vi "Utility Error Query.vi"(5 "Retry Attempts (0)":i32 min=0, 8 "error in (no error)":errorcluster, 11 "VISA resource name":refnum<visa-resource-name>) -> (0 "error out":errorcluster, 1 "Error Message":string, 2 "Error Code":i32[](array[numeric]), 3 "VISA resource name out":refnum<visa-resource-name>)   [LabVIEW 2020, in "ChromTech Series I Drivers.lvlib"]
doc: "Queries the instrument for any errors in the instrument's error queue. It will continue to read errors until all errors have been read from the instrument. Any errors will be returned in the <B>error out</B> control.\n\n<B>Note:</B>\nThis VI is called automatically by most driver VIs so it is not usually necessary to call this in an application."
uses:
  <instrlib>/RxnRover/ChromtechSeriesIDriver/ChromTech Series I Drivers.lvlib
panel:
  # "THIS IS NOT COMPLETE"
  # "EDIT: Note: The Error Query VI is included as a subVI in all driver VIs except low-level API VIs. If the instrument does not support error query, then remove the VI and remove subVI calls in each instrument driver VI that calls it."
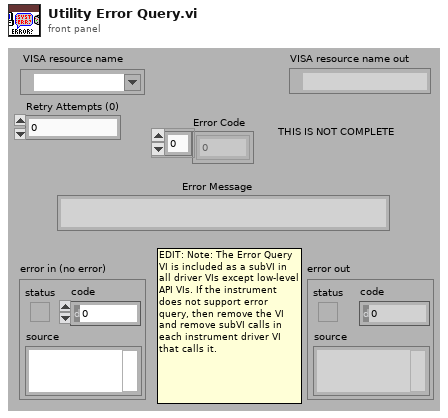
[diagram p1: front panel]
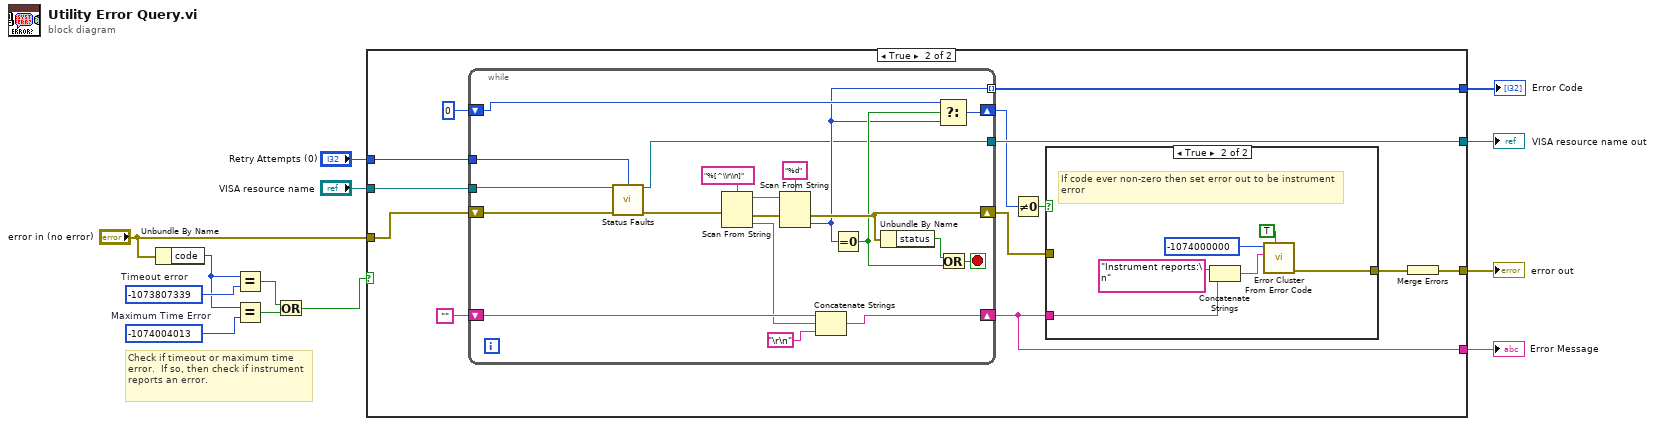
[diagram p0: block diagram]
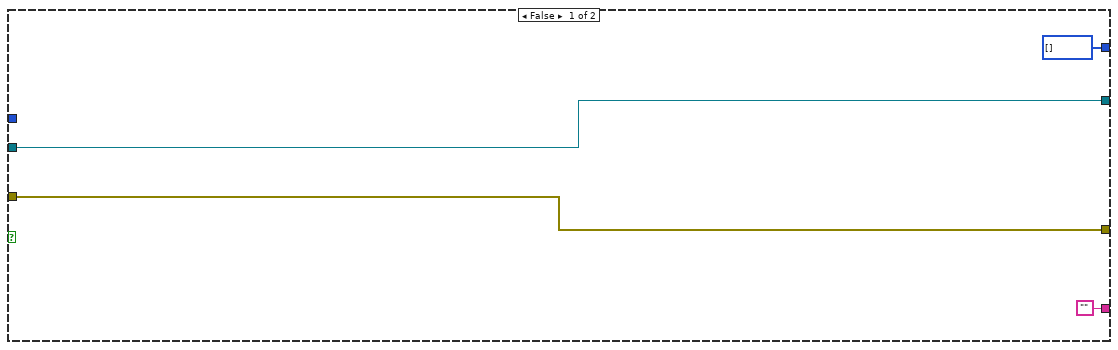
[diagram p2: hidden frame]
diagram:
  w6 = -1074004013  # Maximum Time Error
  w8 = -1073807339  # Timeout error
  # "Check if timeout or maximum time error.  If so, then check if instrument reports an error."
  n1 = Unbundle By Name("error in (no error)") -> ("code"=w7:i32)
  n2 = Equal?(x=w7, y=w8) -> (x = y?=w4:bool)
  n3 = Equal?(x=w7, y=w6) -> (x = y?=w5:bool)
  n4 = Or(x=w4, y=w5) -> (x .or. y?=w2:bool)
  n5 = case shown="True" w2 {
    tunnel: [w17 w30] -> w13
    tunnel: "VISA resource name" -> [w17 w29]
    tunnel: [w14 w27] -> w12
    tunnel: ["" w22] -> w11
    tunnel: [i32[] [] w21] -> w10
    tunnel: "error in (no error)" -> [w14 w19]
    tunnel: "Retry Attempts (0)" -> [_ w18]
    frame False {
    }
    frame True {
      n6 = while {
        tunnel: [w39] -> w30
        tunnel: w29 -> [w40]
        shift-right: [w50] -> w22
        shift-left: "" -> [w53]
        shift-right: [w48] -> w23
        shift-left: 0 -> [w49]
        shift-right: [w46] -> w20
        shift-left: w19 -> [w47]
        tunnel: [w42] -> w21 mode=indexing
        tunnel: w18 -> [w38]
        stop <- w56 stop-if-true
        n7 = call <instrlib>:"Status Faults.vi"("VISA resource name"=w40, "Retry Attempts (0)"=w38, "error in (no error)"=w47) -> ("VISA resource name out"=w39:refnum<visa-resource-name>, "error out"=w41:errorcluster)  [unwired: 8 in, 3 out]
        n8 = Scan From String(format string="%[^\\r\\n]", input string=w54, error in=w41) -> (error out=w45:errorcluster, output 1=w51:string)  [unwired: 2 in, 2 out]
        n9 = Scan From String(format string="%d", error in=w45) -> (input string=w54:string, error out=w46:errorcluster, output 1=w42:i32)  [unwired: 2 in, 2 out]
        n10 = Concatenate Strings(w53, w51, "\r\n") -> (w50:string)
        n11 = Equal To 0?(x=w42) -> (x = 0?=w43:bool)
        n12 = Unbundle By Name(w46) -> ("status"=w44:bool)
        n13 = Select(t=w49, s=w43, f=w42) -> (s? t:f=w48:i32)
        n14 = Or(x=w44, y=w43) -> (x .or. y?=w56:bool)
      }
      n15 = Not Equal To 0?(x=w23) -> (x != 0?=w25:bool)
      n16 = case shown="True" w25 {
        tunnel: w22 -> [_ w36]
        tunnel: [w31 w32] -> w24
        tunnel: w20 -> [w31 _]
        frame False {
        }
        frame True {
          # "If code ever non-zero then set error out to be instrument error"
          n17 = Concatenate Strings("Instrument reports:\n" ("Source"), w36) -> (w33:string)
          n18 = call <vilib>:"Error Cluster From Error Code.vi"("show call chain? (False)"=TRUE, "error message (\"\")"=w33, "error code (0)"=-1074000000 ("Code")) -> ("error out"=w32:errorcluster)  [unwired: 6 in]
        }
      }
      n19 = Merge Errors(w24) -> (w27:errorcluster)
    }
  }
  "VISA resource name out" <- w13
  "error out" <- w12
  "Error Message" <- w11
  "Error Code" <- w10
